vi "Backspace.vi"(8 "error in (no error)":errorcluster, 9 "Display In":ext, 10 "Decimal Count In":u8) -> (0 "error out":errorcluster, 1 "Display Out":ext, 2 "Decimal Count Out":u8)   [LabVIEW 2014]
doc: "This VI handles the backspacing of a decimal number. The way it works is as follows:\n\nThe display is multiplied by 10 raised to however many decimals it has to make it a whole number (ex: 12.34 * 10^2 = 1234).\nNext, we Mod 10 the display (ex: 1234 = 123).\nFinally, we divide the display by the 10 raised to the number of decimals it had minus one (ex: 123 / 10^1 = 12.3)\n\nAuthor: Erik Johnson, National Instruments"
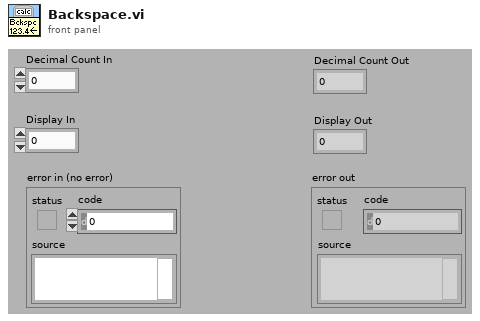
[diagram p1: front panel]
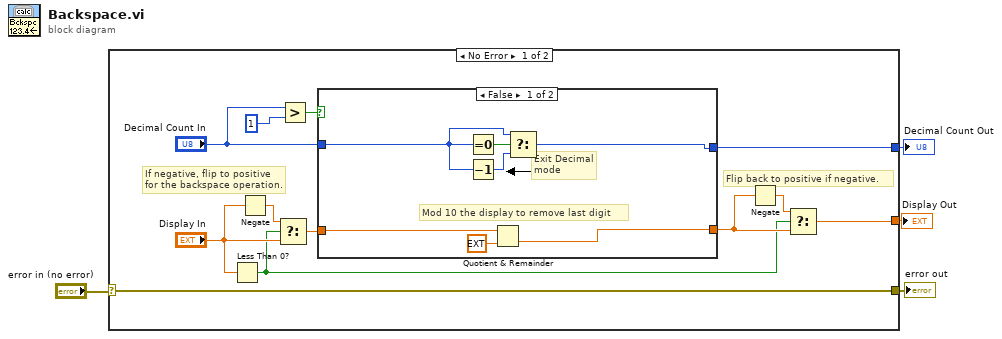
[diagram p0: block diagram]
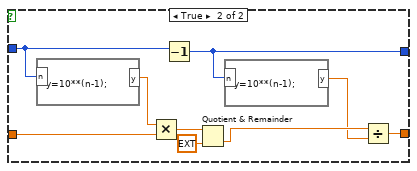
[diagram p2: hidden frame]
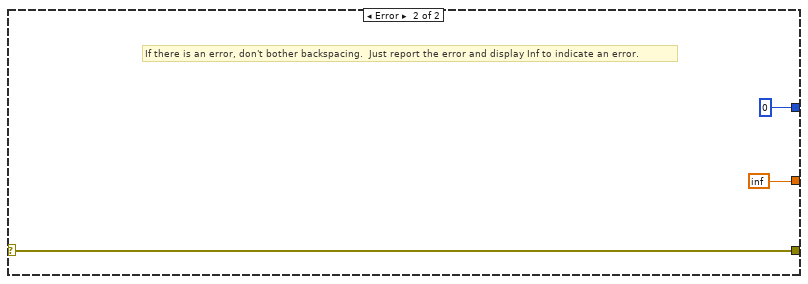
[diagram p3: hidden frame]
diagram:
  n1 = case shown="No Error" "error in (no error)" {
    selector: "error in (no error)" -> [w5 w33]
    tunnel: [w16 u8 0 ("Decimal Count In")] -> w4
    tunnel: [w6 inf] -> w3
    tunnel: [w5 w33] -> w1
    frame No Error {
      # "Flip back to positive if negative."
      # "If negative, flip to positive for the backspace operation."
      n2 = Less Than 0?(x="Display In") -> (x < 0?=w7:bool)
      n3 = Negate(x="Display In") -> (-x=w12:ext)
      n4 = Select(t=w12, s=w7, f="Display In") -> (s? t:f=w10:ext)
      n5 = Greater?(x="Decimal Count In", y=u8 1) -> (0:w13:bool)
      n6 = case shown="False" w13 {
        tunnel: [w19 w32] -> w8
        tunnel: w10 -> [w20 w27]
        tunnel: "Decimal Count In" -> [w21 w26]
        tunnel: [w18 w25] -> w16
        frame False {
          # "Exit Decimal mode"
          # "Mod 10 the display to remove last digit"
          n7 = Equal To 0?(x=w21) -> (x = 0?=w23:bool)
          n8 = Decrement(x=w21) -> (x-1=w22:u8)
          n9 = Quotient & Remainder(x=w20, y=ext 10.0) -> (floor(x/y)=w19:ext)  [unwired: 1 out]
          n10 = Select(t=w21, s=w23, f=w22) -> (s? t:f=w18:u8)
        }
        frame True {
          n11 = formula code="y=10**(n-1);"("n"=w26) -> ("y"=w28:dbl)
          n12 = Multiply(x=w28, y=w27) -> (x*y=w29:ext)
          n13 = Decrement(x=w26) -> (x-1=w25:u8)
          n14 = Quotient & Remainder(x=w29, y=ext 10.0) -> (floor(x/y)=w31:ext)  [unwired: 1 out]
          n15 = formula code="y=10**(n-1);"("n"=w25) -> ("y"=w24:dbl)
          n16 = Divide(x=w31, y=w24) -> (x/y=w32:ext)
        }
      }
      n17 = Negate(x=w8) -> (-x=w9:ext)
      n18 = Select(t=w9, s=w7, f=w8) -> (s? t:f=w6:ext)
    }
    frame Error {
      # "If there is an error, don't bother backspacing.  Just report the error and display Inf to indicate an error."
    }
  }
  "Display Out" <- w3
  "Decimal Count Out" <- w4
  "error out" <- w1
